vi "Calculate Wavelengths (Full Sensor).vi"(10 "Numeric":i32, 11 "Polynomial Coefficients in":dbl[](array[numeric])) -> (2 "wavelengths":dbl[](array[numeric]), 3 "Polynomial Coefficients":dbl[](array[numeric]))   [LabVIEW 2019, in "Spectrometer Calibration.lvlib"]
uses:
  Spectrometer Calibration.lvlib
  <vilib>/Analysis/1siggen.llb/Ramp Pattern by Samples.vi
  <vilib>/Analysis/polynomials.llb/1D Polynomial Evaluation (DBL).vi
  <vilib>/Analysis/NI_AALPro.lvlib
  <vilib>/Analysis/NI_AALBase.lvlib
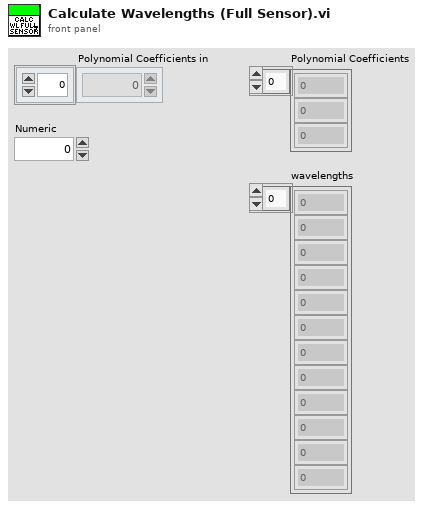
[diagram p1: front panel]
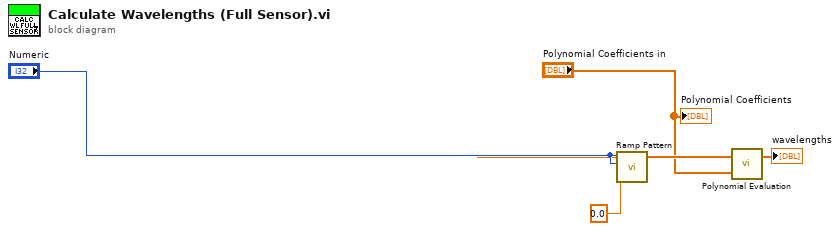
[diagram p0: block diagram]
diagram:
  n1 = call-poly <vilib>:"Ramp Pattern.vi"("start"=0.0, "end"="Numeric", "samples"="Numeric") -> ("Ramp Pattern"=w3:dbl[])  [unwired: 7 in, 1 out]
  n2 = call-poly <vilib>:"Polynomial Evaluation.vi"("P(x)"="Polynomial Coefficients in", "A"=w3) -> ("P(A)"=→"wavelengths":dbl[])  [unwired: 1 out]
  "Polynomial Coefficients" <- "Polynomial Coefficients in"
